vi "Analog Output Waveform.vi"(8 "error in (no error)":errorcluster, 10 "Waveform Generation":T1(array[cluster]), 11 "NI Waveform Output in":refnum<class "NI Waveform Output.lvclass">) -> (0 "error out":errorcluster, 3 "NI Waveform Output out":refnum<class "NI Waveform Output.lvclass">)   [LabVIEW 2023, in "HardwareAbstractionLayer_LVOOP.lvlib" / "NI Waveform Output.lvclass"]
uses:
  NI Waveform Output.lvclass
  NI Waveform Output.lvclass/NI Waveform Output.ctl
  <vilib>/DAQmx/write.llb/DAQmx Write (Analog 1D Wfm NChan NSamp).vi
  <vilib>/DAQmx/miscellaneous.llb/DAQmx Fill In Error Info.vi
  <vilib>/measure/NI_MABase.lvlib
  <resource>/objmgr/daqmx.rc
panel:
  out "Waveform Graph":waveform(dbl)[](graph)=[{"t0"=timestamp(0 s since 1904-01-01), "dt"=0.001, "Y"=[]}]
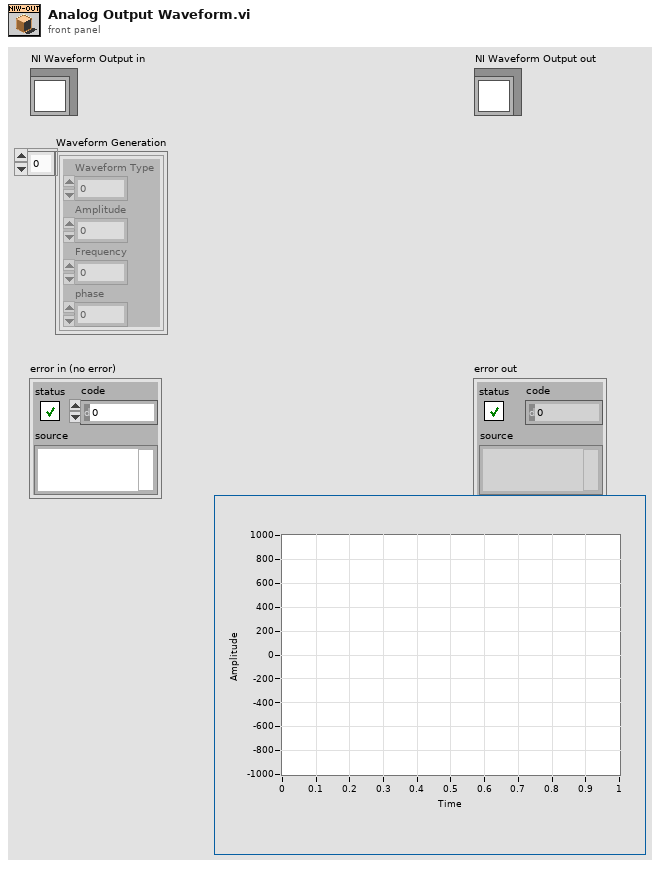
[diagram p1: front panel]
types:
  T1 = cluster{"Waveform Type":u16, "Amplitude":dbl, "Frequency":dbl, "phase":dbl}[]
  T2 = enum16{"Sine Wave", "Triangle Wave", "Square Wave", "Sawtooth Wave"}
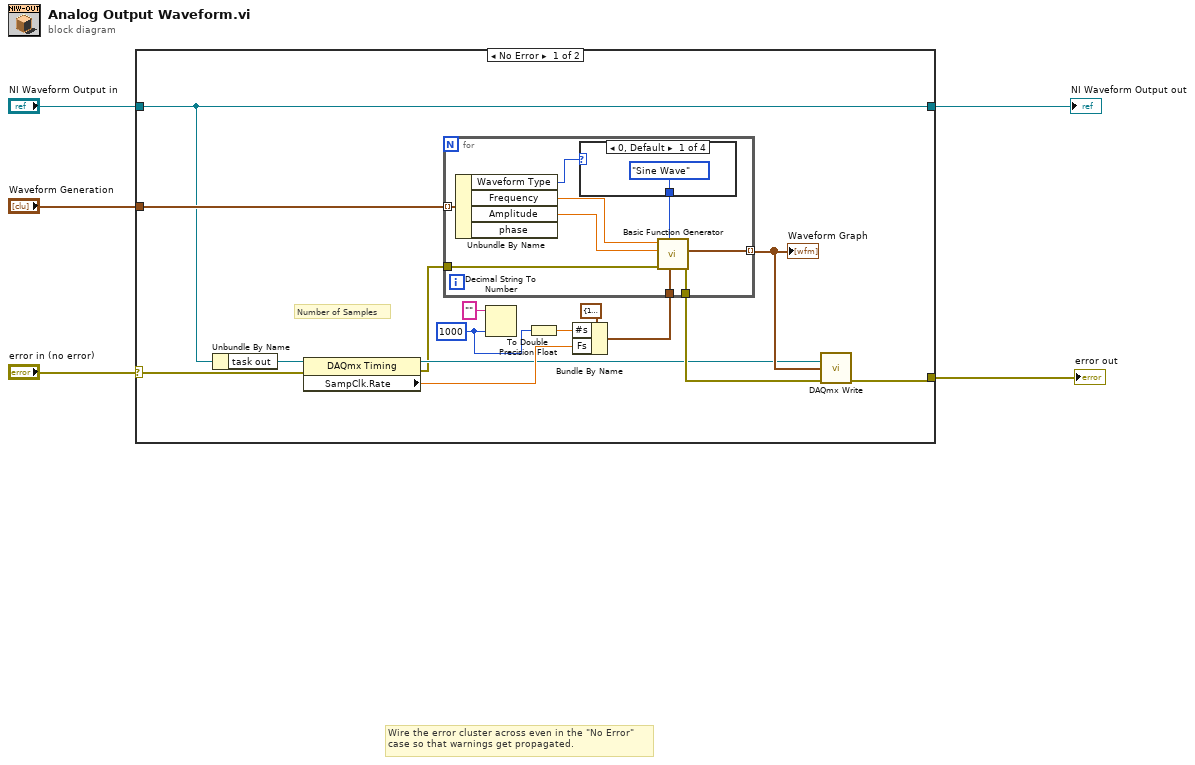
[diagram p0: block diagram]
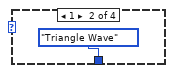
[diagram p2: hidden frame]
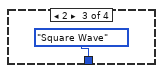
[diagram p3: hidden frame]
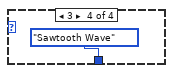
[diagram p4: hidden frame]
diagram:
  # "Wire the error cluster across even in the \"No Error\"\ncase so that warnings get propagated."
  n1 = case shown="No Error" "error in (no error)" {
    selector: "error in (no error)" -> [w9 w35]
    tunnel: [w8 w35] -> w4
    tunnel: [w11 w34] -> w2
    tunnel: "NI Waveform Output in" -> [w11 w34]
    tunnel: "Waveform Generation" -> [w12 _]
    frame No Error {
      w6 = 1000 ("Number of Samples")
      # "Number of Samples"
      n2 = Unbundle By Name(w11) -> ("task out"=w10:refnum<k21>)
      n3 = property class="DAQmx Timing"(reference=w10, error in=w9) -> (reference out=w14:refnum<k21>, error out=w13:errorcluster, "SampClk.Rate"=w15:dbl)
      n4 = Decimal String To Number(string="", default (0L)=w6) -> ()  [unwired: 1 in, 2 out]
      n5 = To Double Precision Float(number=w6) -> (double precision float=w16:dbl)
      n6 = Bundle By Name(cluster=cluster{"Fs":dbl, "#s":dbl} {"Fs"=1000.0, "#s"=1000.0} ("sampling info"), "#s"=w16, "Fs"=w15) -> (w19:cluster{"Fs":dbl, "#s":dbl})
      n7 = for {
        tunnel: w19 -> [w29]
        tunnel: [w28] -> w18
        tunnel: w12 -> [w27] mode=indexing
        tunnel: [w24] -> w17 mode=indexing
        tunnel: w13 -> [w23]
        n8 = Unbundle By Name(w27) -> ("Waveform Type"=w22:u16, "Frequency"=w26:dbl, "Amplitude"=w25:dbl)  [unwired: 1 out]
        n9 = case shown="0, Default" w22 {
          tunnel: [T2."Sine Wave" ("signal type") T2."Triangle Wave" ("signal type") T2."Square Wave" ("signal type") T2."Sawtooth Wave" ("signal type")] -> w21
          frame 0, Default {
          }
          frame 1 {
          }
          frame 2 {
          }
          frame 3 {
          }
        }
        n10 = call <vilib>:"Basic Function Generator.vi"("sampling info"=w29, "signal type"=w21, "error in (no error)"=w23, "amplitude"=w25, "frequency"=w26) -> ("error out"=w28:errorcluster, "signal out"=w24:waveform(dbl))  [unwired: 4 in, 1 out]
      }
      "Waveform Graph" <- w17
      n11 = call-poly <vilib>:"DAQmx Write.vi"("task/channels in"=w14, "data"=w17, "error in"=w18) -> ("error out"=w8:errorcluster)  [unwired: 10 in, 2 out]
    }
    frame Error {
    }
  }
  "error out" <- w4
  "NI Waveform Output out" <- w2
